vi "Get Credentials.vi"() -> (3 "Azure Credentials":T1)   [LabVIEW 2015, in "_Unit Tests Shared.lvlib"]
uses:
  _Unit Tests Shared.lvlib
  Core/Azure Credentials.ctl
  Core/NI_Azure_Core.lvlib
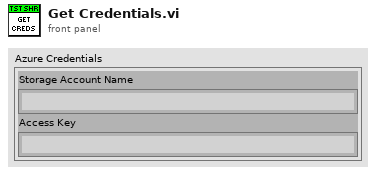
[diagram p1: front panel]
types:
  T1 = typedef "NI_Azure_Core.lvlib/Azure Credentials.ctl" = cluster{"Storage Account Name":string, "Access Key":string}
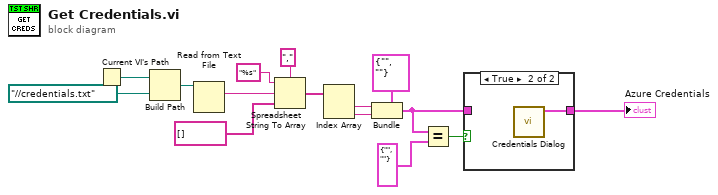
[diagram p0: block diagram]
diagram:
  n1 = Current VI's Path() -> (path=w2:path)
  n2 = Build Path(base path=w2, name or relative path=path "../../credentials.txt") -> (appended path=w4:path)
  n3 = Read from Text File(file (use dialog)=w4) -> (text=w6:string)  [unwired: 3 in, 3 out]
  n4 = Spreadsheet String To Array(delimiter (Tab)=",", format string="%s", spreadsheet string=w6, array type (2D Dbl)=string[] []) -> (array=w9:string[])
  n5 = Index Array(array=w9) -> (element #1=w10:string, element #2=w11:string)  [unwired: 2 in]
  n6 = Bundle(cluster=T1 {"Storage Account Name"="", "Access Key"=""} ("Azure Credentials out"), "Storage Account Name"=w10, "Access Key"=w11) -> (w14:T1)
  n7 = Equal?(x=w14, y=T1 {"Storage Account Name"="", "Access Key"=""}) -> (x = y?=w15:bool)
  n8 = case shown="True" w15 {
    tunnel: [w16 w17] -> w1
    tunnel: w14 -> [w16 _]
    frame False {
    }
    frame True {
      n9 = call "Credentials Dialog.vi"() -> ("Azure Credentials out"=w17:T1)  [unwired: 11 in]
    }
  }
  "Azure Credentials" <- w1
